vi "Read Property.vi"(6 "timeout (ms)":i32=-1, 8 "error in (no error)":errorcluster, 10 "property name":string, 11 "FlexLogger_gRPCAPI in":refnum<class "FlexLogger_gRPC.lvclass">) -> (0 "error out":errorcluster, 2 "Test_Properties Array":T1, 3 "FlexLogger_gRPCAPI out":refnum<class "FlexLogger_gRPC.lvclass">)   [LabVIEW 2020, in "FlexLogger_gRPC.lvlib" / "FlexLogger_gRPC.lvclass"]
doc: "Gets a specific test property of currently opened project in flexlogger"
uses:
  FlexLogger_gRPC.lvclass
  Controls/test_property Type.ctl
  FlexLogger_client/RPC Messages/flexlogger_GetTestPropertyRequest.ctl
  FlexLogger_client/RPC Messages/flexlogger_ElementIdentifier.ctl
  FlexLogger_gRPC.lvclass/FlexLogger_gRPC.ctl
  FlexLogger_client/FlexLogger_client.lvlib
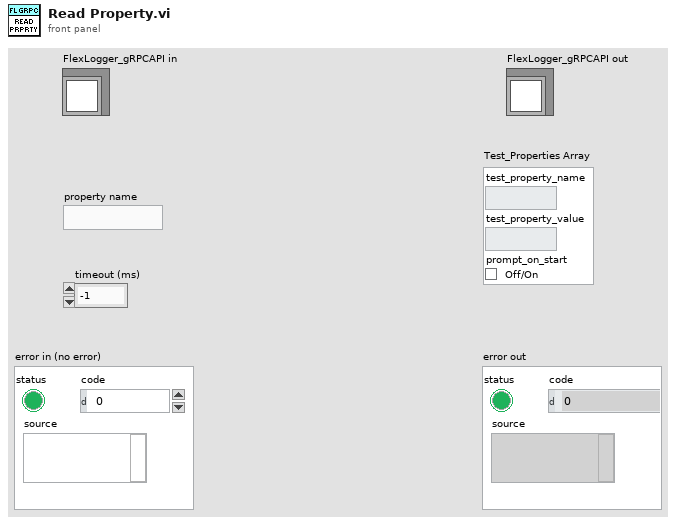
[diagram p1: front panel]
types:
  T1 = typedef "FlexLogger_gRPC.lvlib/FlexLogger_gRPC.lvclass/test_property Type.ctl" = cluster{"test_property_name":string, "test_property_value":string, "prompt_on_start":bool}
  T2 = typedef "FlexLogger_client.lvlib/flexlogger_GetTestPropertyRequest.ctl" = cluster{"document_identifier":T3, "property_name":string}
  T3 = typedef "FlexLogger_client.lvlib/flexlogger_ElementIdentifier.ctl" = cluster{"project_id":string, "file_name":string, "element_id":string, "subpart_id":string}
  T4 = typedef "grpc-lvsupport-release.lvlib/grpcId.ctl" = u64
  T5 = typedef "FlexLogger_client.lvlib/flexlogger_GetTestPropertyResponse.ctl" = cluster{"test_property":T6}
  T6 = typedef "FlexLogger_client.lvlib/flexlogger_TestProperty.ctl" = cluster{"property_name":string, "property_value":string, "prompt_on_start":bool}
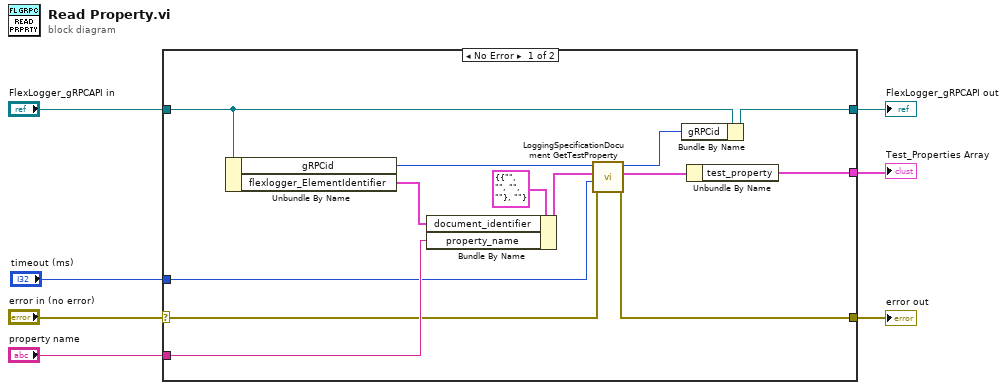
[diagram p0: block diagram]
diagram:
  n1 = case shown="No Error" "error in (no error)" {
    selector: "error in (no error)" -> [w10 w21]
    tunnel: [w20 _] -> w5
    tunnel: "FlexLogger_gRPCAPI in" -> [w19 w22]
    tunnel: [w18 w22] -> w6
    tunnel: [w16 w21] -> w4
    tunnel: "property name" -> [w12 _]
    tunnel: "timeout (ms)" -> [w8 _]
    frame No Error {
      n2 = Unbundle By Name(w19) -> ("gRPCid"=w11:T4, "flexlogger_ElementIdentifier"=w9:T3)
      n3 = Bundle By Name(cluster=T2 {"document_identifier"={"project_id"="", "file_name"="", "element_id"="", "subpart_id"=""}, "property_name"=""} ("Request Data"), "document_identifier"=w9, "property_name"=w12) -> (w13:T2)
      n4 = call "LoggingSpecificationDocument GetTestProperty.vi"("error in"=w10, "timeout (ms)"=w8, "Request Data"=w13, "gRPC ID"=w11) -> ("error out"=w16:errorcluster, "Response Data"=w15:T5, "gRPC ID out"=w17:T4)  [unwired: 5 in]
      n5 = Bundle By Name(cluster=w19, "gRPCid"=w17) -> (w18:refnum<class "FlexLogger_gRPC.lvclass">)
      n6 = Unbundle By Name(w15) -> ("test_property"=w20:T6)
    }
    frame Error {
    }
  }
  "error out" <- w4
  "FlexLogger_gRPCAPI out" <- w6
  "Test_Properties Array" <- w5
